vi "Get_Number_Of-Problem_Points_in_Group-1.vi"(1 "[IN] Dot Statuses":i16[][](array[numeric])) -> (0 "[OUT] Number of problem points":i32)   [LabVIEW 2013]
doc: "The SubVI estimates number of points with problems as condition for starting the resolving correspondence problems"
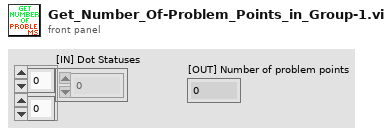
[diagram p1: front panel]
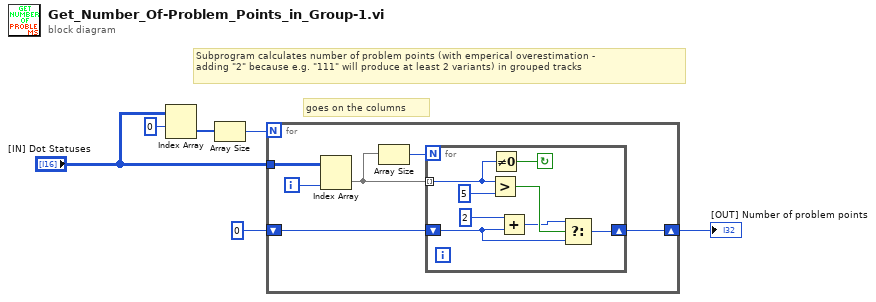
[diagram p0: block diagram]
diagram:
  # "Subprogram calculates number of problem points (with emperical overestimation - \nadding \"2\" because e.g. \"111\" will produce at least 2 variants) in grouped tracks"
  # "goes on the columns"
  n1 = Index Array(array="[IN] Dot Statuses", index (row)=0) -> (element=w5:i16[])  [unwired: 1 in]
  n2 = Array Size(array=w5) -> (size(s)=w4:i32)
  n3 = for {
    N: w4 -> [_]
    tunnel: "[IN] Dot Statuses" -> [w12]
    shift-right: [w7] -> w1
    shift-left: 0 -> [w8]
    i -> [w11]
    n4 = Index Array(array=w12, index (col)=w11) -> (element=w9:i16[])  [unwired: 1 in]
    n5 = Array Size(array=w9) -> (size(s)=w10:i32)
    n6 = for {
      N: w10 -> [_]
      tunnel: w9 -> [w19] mode=indexing
      shift-right: [w17] -> w7
      shift-left: w8 -> [w14]
      stop <- w18 continue-if-true
      n7 = Greater?(x=w19, y=i16 5) -> (0:w16:bool)
      n8 = Not Equal To 0?(x=w19) -> (x != 0?=w18:bool)
      n9 = Add(x=2, y=w14) -> (x+y=w15:i32)
      n10 = Select(t=w15, s=w16, f=w14) -> (s? t:f=w17:i32)
    }
  }
  "[OUT] Number of problem points" <- w1
